vi ".NET SubItem Information to G Datatype Child Information.vi"(8 "error in (no error)":errorcluster, 9 ".NET AdsSubItem":refnum<k24>, 11 "TwinCAT ADS in":refnum<class "TwinCAT ADS.lvclass">) -> (0 "error out":errorcluster, 2 "Datatype Child Information":T1 {"Category" items=["Unknown, None"=0, "Primitive"=1, "Alias"=2, "Enum"=3, "Array"=4, "Struct"=5, "FunctionBlock"=6, "Program"=7, "Function"=8, "SubRange"=9, "String"=10, "Bitset"=12, "Pointer"=13, "Union"=14, "Reference"=15, "Interface"=16]; "Type ID" items=["ADST_VOID"=0, "ADST_INT16"=2, "ADST_INT32"=3, "ADST_REAL32"=4, "ADST_REAL64"=5, "ADST_INT8"=16, "ADST_UINT8"=17, "ADST_UINT16"=18, "ADST_UINT32"=19, "ADST_INT64"=20, "ADST_UINT64"=21, "ADST_STRING"=30, "ADST_WSTRING"=31, "ADST_REAL80"=32, "ADST_BIT"=33, "ADST_MAXTYPES"=34, "ADST_BIGTYPE"=65]}, 3 "TwinCAT ADS out":refnum<class "TwinCAT ADS.lvclass">)   [LabVIEW 2018, in "TwinCAT ADS.lvclass"]
uses:
  TwinCAT ADS.lvclass
  TwinCAT.Ads
  Controls/Datatype Child Information.ctl
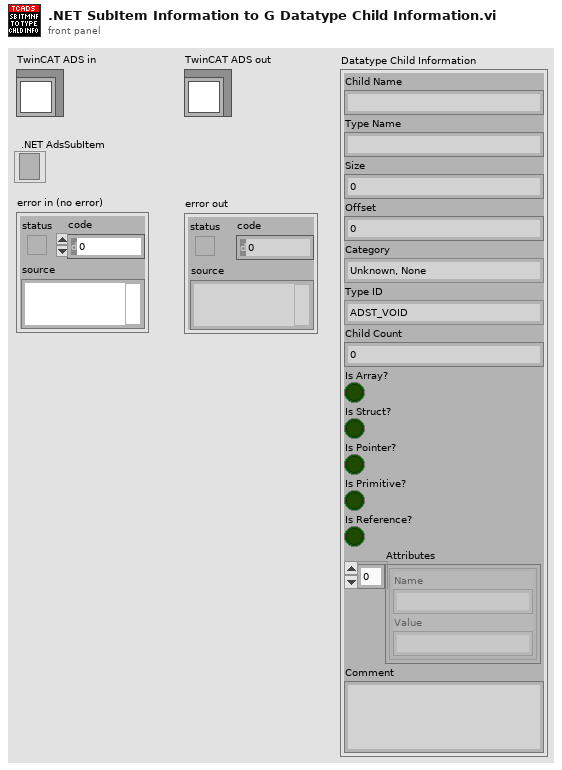
[diagram p1: front panel]
types:
  T1 = typedef "TwinCAT ADS.lvclass/Datatype Child Information.ctl" = cluster{"Child Name":string, "Type Name":string, "Size":i32, "Offset":i32, "Category":i32, "Type ID":i32, "Child Count":i32, "Is Array?":bool, "Is Struct?":bool, "Is Pointer?":bool, "Is Primitive?":bool, "Is Reference?":bool, "Attributes":cluster{"Name":string, "Value":string}[], "Comment":string}
  T2 = typedef "TwinCAT ADS.lvclass/Datatype Information.ctl" = cluster{"Name":string, "Size":i32, "Category":i32, "Type ID":i32, "Child Count":i32, "Is Array?":bool, "Is Struct?":bool, "Is Pointer?":bool, "Is Primitive?":bool, "Is Reference?":bool, "Attributes":cluster{"Name":string, "Value":string}[], "Comment":string}
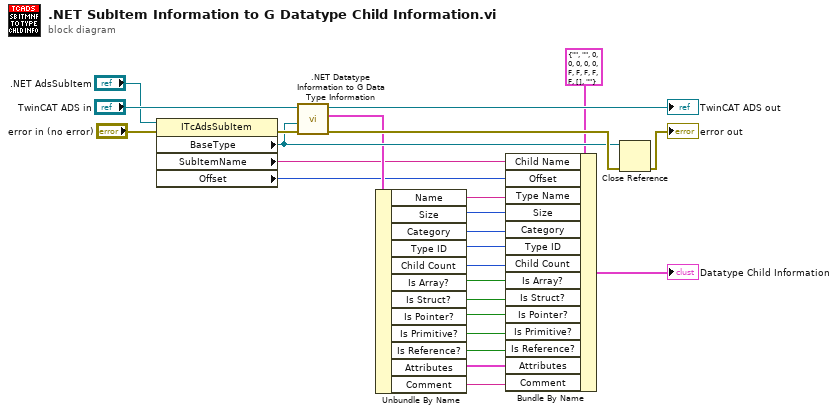
[diagram p0: block diagram]
diagram:
  n1 = property class="ITcAdsSubItem"(reference=".NET AdsSubItem", error in="error in (no error)") -> (error out=w23:errorcluster, "BaseType"=w22:refnum<k24>, "SubItemName"=w15:string, "Offset"=w14:i32)  [unwired: 1 out]
  n2 = call ".NET Datatype Information to G Data Type Information.vi"("error in (no error)"=w23, ".NET Data Type Information"=w22, "TwinCAT ADS in"="TwinCAT ADS in") -> ("error out"=w24:errorcluster, "Data Type Information"=w16:T2, "TwinCAT ADS out"=→"TwinCAT ADS out":refnum<class "TwinCAT ADS.lvclass">)  [unwired: 6 in]
  n3 = Unbundle By Name(w16) -> ("Name"=w13:string, "Size"=w12:i32, "Category"=w11:i32, "Type ID"=w10:i32, "Child Count"=w9:i32, "Is Array?"=w8:bool, "Is Struct?"=w7:bool, "Is Pointer?"=w6:bool, "Is Primitive?"=w5:bool, "Is Reference?"=w4:bool, "Attributes"=w3:cluster{"Name":string, "Value":string}[], "Comment"=w2:string)
  n4 = Bundle By Name(cluster=T1 {"Child Name"="", "Type Name"="", "Size"=0, "Offset"=0, "Category"=0, "Type ID"=0, "Child Count"=0, "Is Array?"=FALSE, "Is Struct?"=FALSE, "Is Pointer?"=FALSE, "Is Primitive?"=FALSE, "Is Reference?"=FALSE, "Attributes"=[], "Comment"=""} ("Data Type Information"), "Child Name"=w15, "Offset"=w14, "Type Name"=w13, "Size"=w12, "Category"=w11, "Type ID"=w10, "Child Count"=w9, "Is Array?"=w8, "Is Struct?"=w7, "Is Pointer?"=w6, "Is Primitive?"=w5, "Is Reference?"=w4, "Attributes"=w3, "Comment"=w2) -> (→"Datatype Child Information":T1)
  n5 = Close Reference(reference=w22, error in (no error)=w24) -> (error out=→"error out":errorcluster)
